vi "PartialClusters3.vi"(3 "Cluster3":T1={"Name3"="", "digital waveform"={"t0"=timestamp(0 s since 1904-01-01), "dt"=0.0, "Y"={"transitions"=[], "data"=[]}, "error"={"status"=FALSE, "code"=37421928, "source"=""}}, "waveform in"={"t0"=timestamp(0 s since 1904-01-01), "dt"=1.0, "Y"=[]}, "Dynamic Data Type"=0.0}, 4 "Cluster2":cluster{"Name2":string}, 5 "Cluster1":T2={"Name1"="", "Cluster1.1"={"ArrayOfNum"=[34.0, 35.0, 36.0]}}) -> (0 "dt":dbl, 1 "element":dbl)   [LabVIEW 2013]
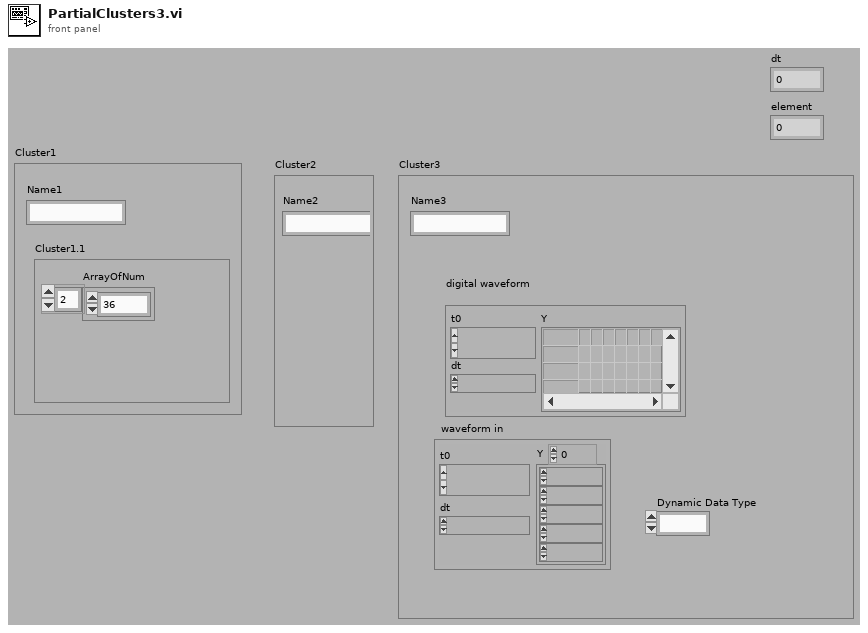
[diagram p1: front panel]
types:
  T1 = cluster{"Name3":string, "digital waveform":digitalwaveform, "waveform in":waveform(dbl), "Dynamic Data Type":dbl}
  T2 = cluster{"Name1":string, "Cluster1.1":cluster{"ArrayOfNum":dbl[]}}
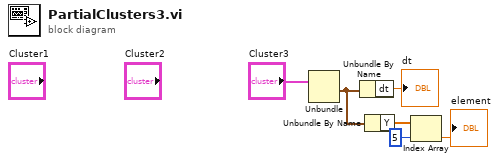
[diagram p0: block diagram]
diagram:
  n1 = Unbundle("Cluster3") -> ("waveform in"=w4:waveform(dbl))  [unwired: 3 out]
  n2 = Unbundle By Name(w4) -> ("dt"=→"dt":dbl)
  n3 = Unbundle By Name(w4) -> ("Y"=w3:dbl[])
  n4 = Index Array(array=w3, index=5) -> (element=→"element":dbl)
